vi "FXP NILIA_PLL.vi"(8 "reset?":bool, 9 "norminal freq [U16.0]":fxp<+,16,0>, 10 "alpha [U16.0]":fxp<+,16,0>, 11 "x[I16.1]":fxp<+/-,16,1>) -> (0 "f":fxp<+/-,32,0> format="%.32g", 1 "z [I32.1]":fxp<+/-,32,1>, 2 "sin(z)":fxp<+/-,16,2> format="%.15g", 3 "cos(z)":fxp<+/-,16,2> format="%.15g")   [LabVIEW 2012]
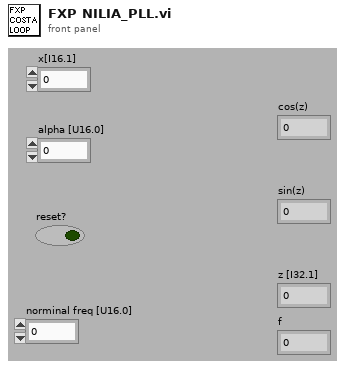
[diagram p1: front panel]
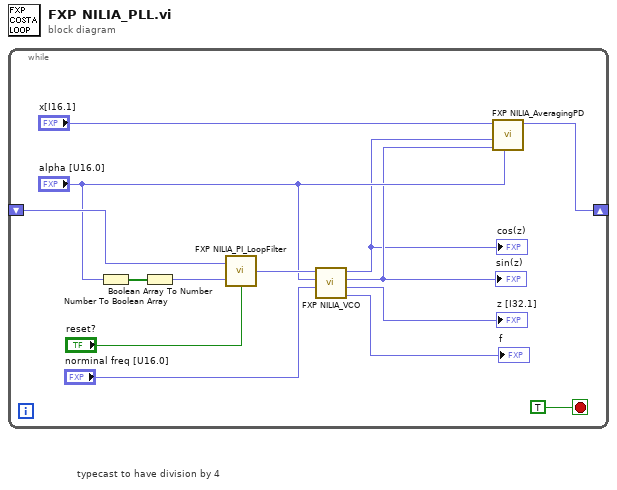
[diagram p0: block diagram]
diagram:
  # "typecast to have division by 4"
  n1 = while {
    shift-right: [w13] -> _
    shift-left: _ -> [w10]
    stop <- TRUE stop-if-true
    n2 = Number To Boolean Array(number="alpha [U16.0]") -> (Boolean array=w8:bool[])
    n3 = Boolean Array To Number(Boolean array=w8) -> (number=w7:fxp<+,16,-2>)
    n4 = call "FXP NILIA_PI_LoopFilter.vi"("reset?"="reset?", "alpha [U16.-2]"=w7, "x [I16.2]"=w10) -> ("x+y [I32.17]"=w12:fxp<+/-,32,17>)
    n5 = call "FXP NILIA_VCO.vi"("nominal freq [U16.0]"="norminal freq [U16.0]", "Kv [U16.0]"="alpha [U16.0]", "v [I32.17]"=w12) -> ("f"=→"f":fxp<+/-,32,0>, "z [I32.1]"=→"z [I32.1]":fxp<+/-,32,1>, "sin(z) [I16.2]"=w3:fxp<+/-,16,2>, "cos(z) [I16.2]"=w2:fxp<+/-,16,2>)  [unwired: 5 out]
    "sin(z)" <- w3
    "cos(z)" <- w2
    n6 = call "FXP NILIA_AveragingPD.vi"("alpha [U16.0]"="alpha [U16.0]", "sin(z) [I16.2]"=w3, "cos(z) [I16.2]"=w2, "x[I16.1]"="x[I16.1]") -> ("psd_out"=w13:fxp<+/-,16,2>)  [unwired: 7 out]
  }
